vi "report_view.vi"   [LabVIEW 2025]
uses:
  <vilib>/Utility/TDMS File Viewer/NI_TDMS File Viewer.lvlib
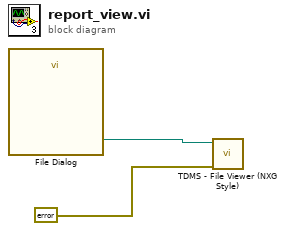
[diagram p0: block diagram]
diagram:
  n1 = call "File Dialog"() -> ("selected path"=w2:path)  [unwired: 12 in, 3 out]
  n2 = call <vilib>:"TDMS - File Viewer (NXG Style).vi"("error in"=errorcluster {"status"=FALSE, "code"=0, "source"=""}, "file in"=w2) -> ()  [unwired: 8 in, 2 out]
